vi "Main.vi"() -> ()   [LabVIEW 2019]
uses:
  <vilib>/vision/Image Controls.llb/IMAQ Image.ctl
  <vilib>/vision/NI_Vision_Development_Module.lvlib
panel:
  out "Otwarte":bool
  in  "Save Button":bool
  in  "Clear Button":bool
  in  "Image Path":path=path "D:/Krystian/Krystian/LabVIEW Data/OSP Projekt/Data/(0).jpg" caption="Picture Path"
  in  "Exit":bool
  in  "Start":bool
  out "Results":string
  out "Image":T1(plugin-control)
  # "Application Panel"
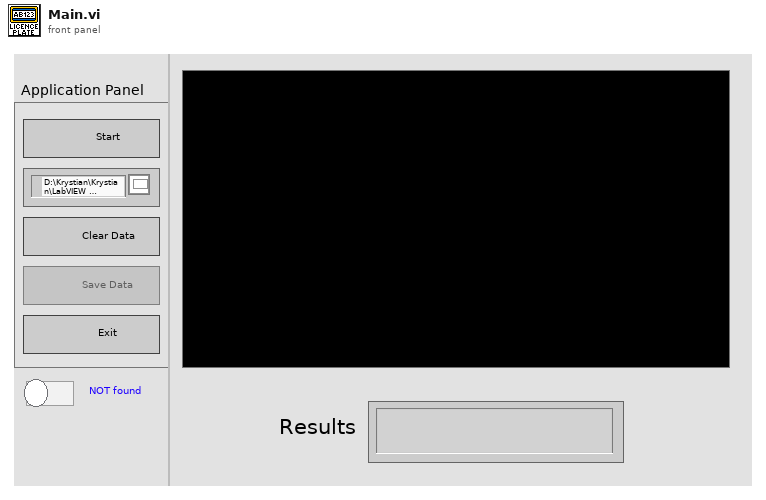
[diagram p1: front panel]
types:
  T1 = typedef "IMAQ Image.ctl" = refnum<image>
  T2 = enum32{"Invalid", "Standard", "Closed", "Hidden", "Minimized", "Maximized"}
  T3 = enum32{"invalid app kind", "Development System", "Run Time System", "Student Edition", "Embedded LabVIEW", "Evaluation", "Custom"}
  T4 = enum8{"Enabled", "Disabled", "Disabled and Grayed Out"}
  T5 = cluster{"Core":cluster{"Current VI Reference":refnum<vi>, "Close Panel on Exit?":bool}, "Save Button":refnum<vi>, "Results":string, "Image Path":path, "Data":cluster{"Rectangle":i32[]}, "Image":refnum<image>, "Python Path":path}
  T6 = cluster{"Current VI Reference":refnum<vi>, "Close Panel on Exit?":bool}
  T7 = typedef "Image Type" = u32
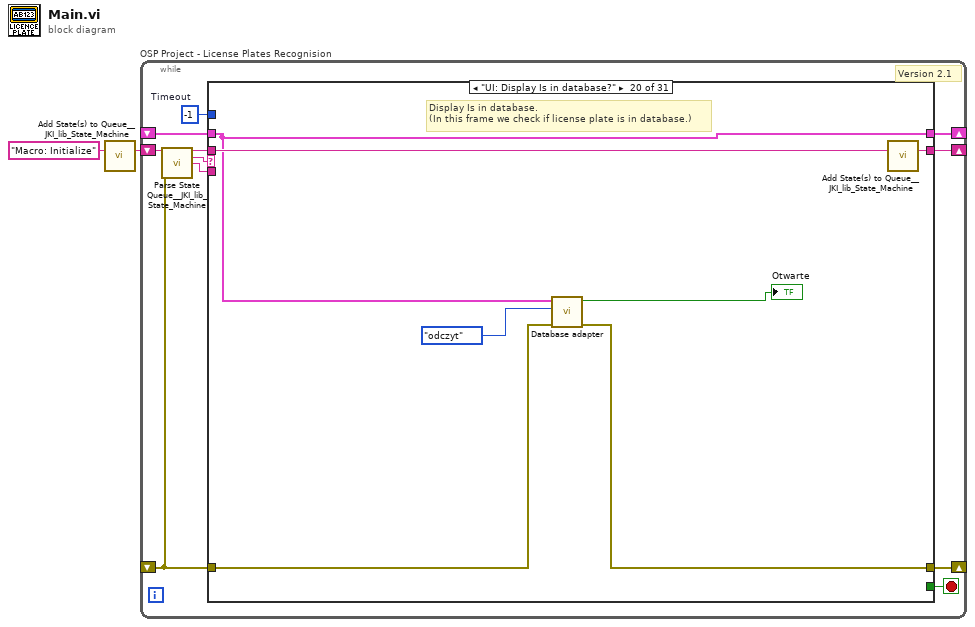
[diagram p0: block diagram]
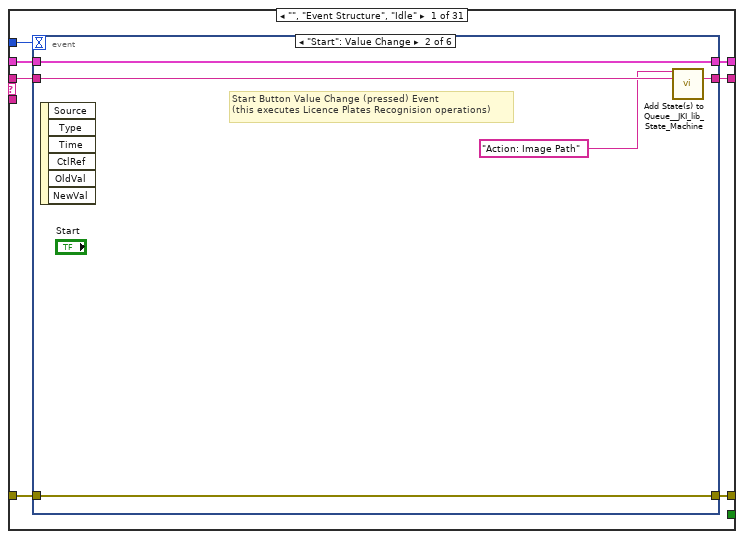
[diagram p2: hidden frame]
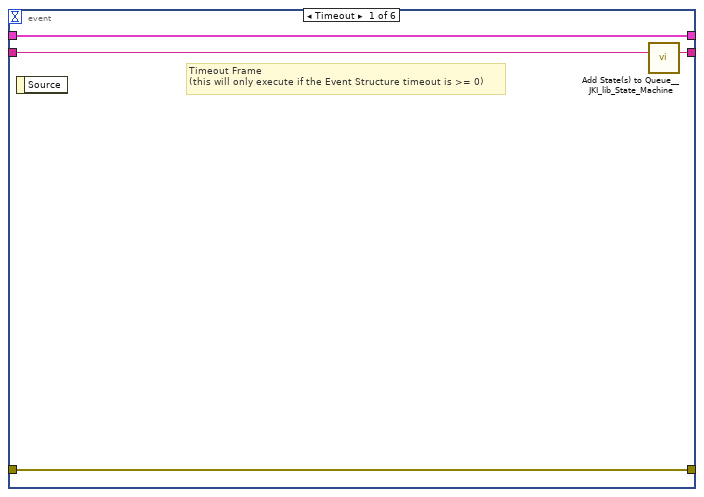
[diagram p3: hidden frame]
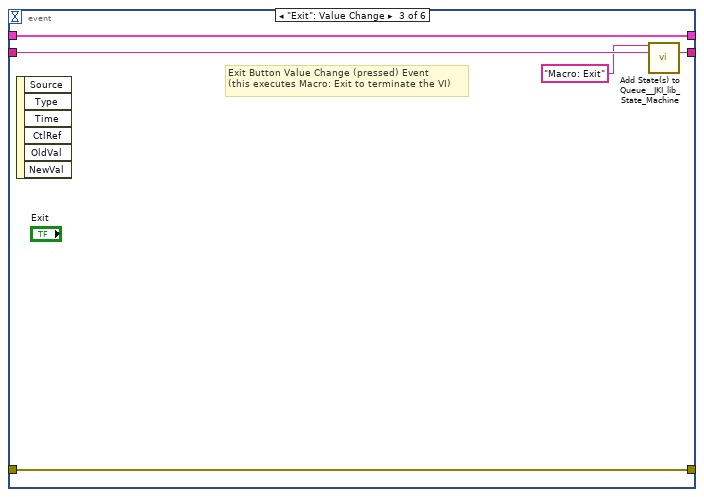
[diagram p4: hidden frame]
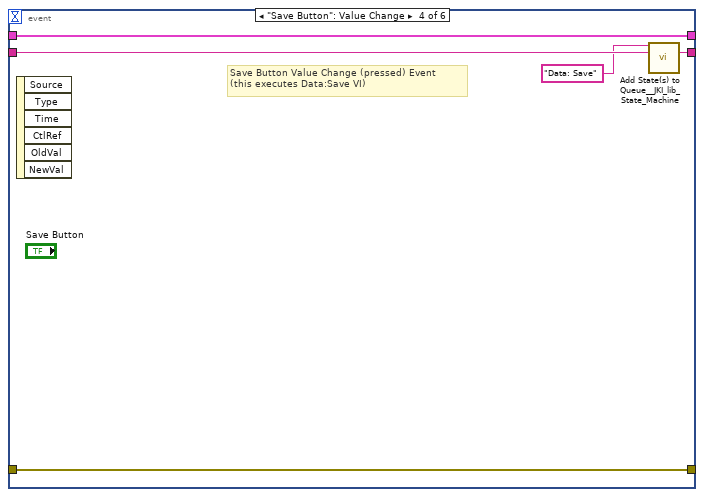
[diagram p5: hidden frame]
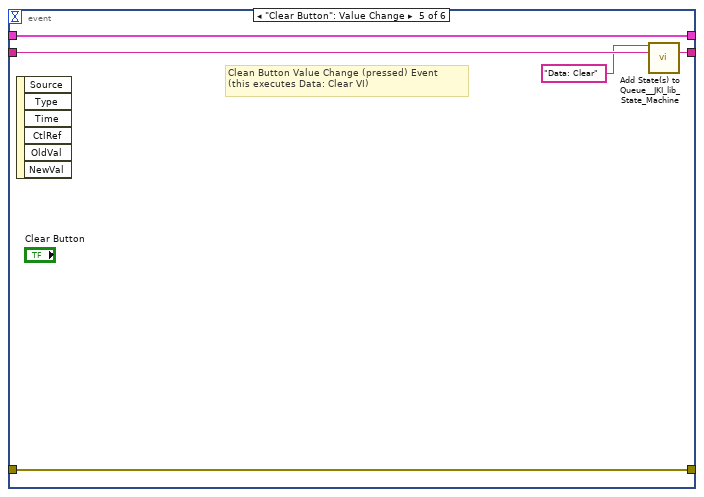
[diagram p6: hidden frame]
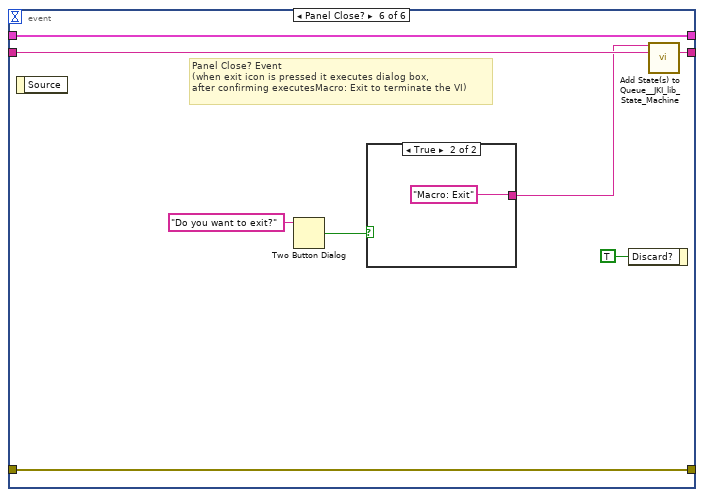
[diagram p7: hidden frame]
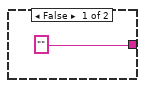
[diagram p8: hidden frame]
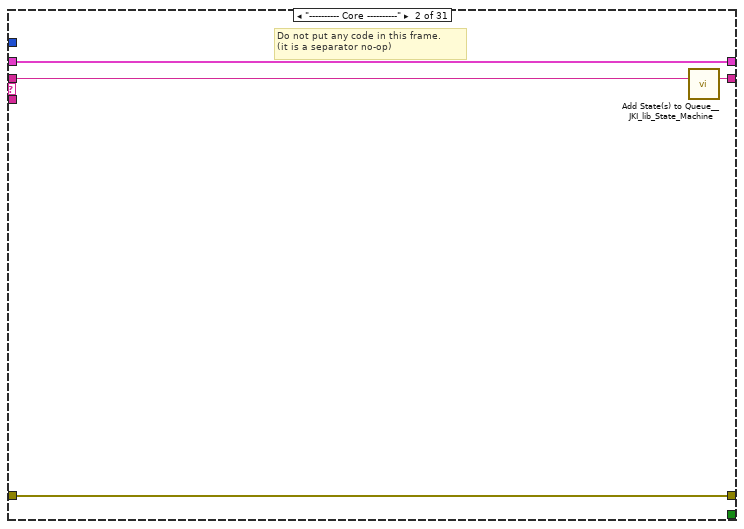
[diagram p9: hidden frame]
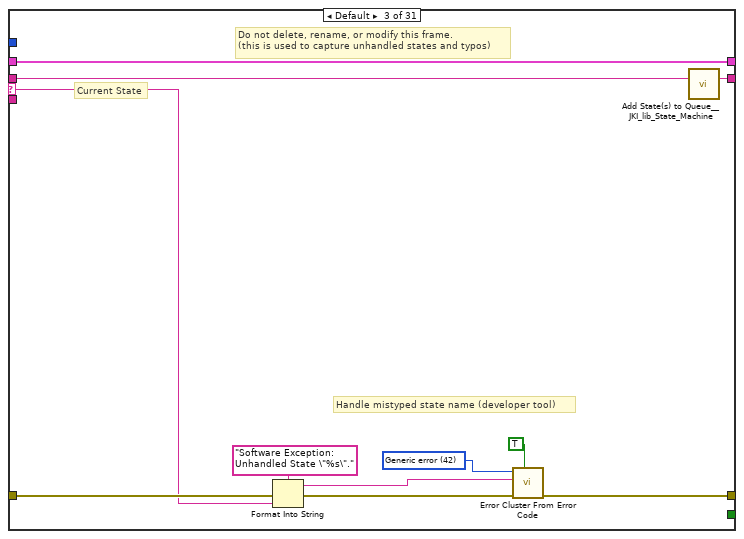
[diagram p10: hidden frame]
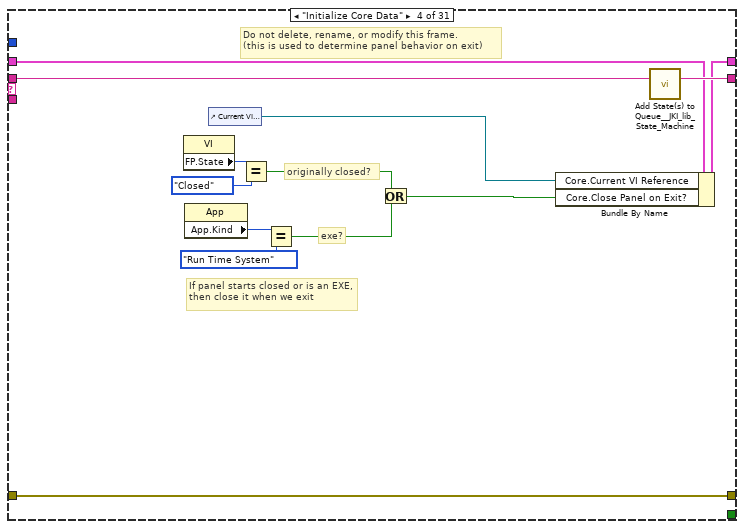
[diagram p11: hidden frame]
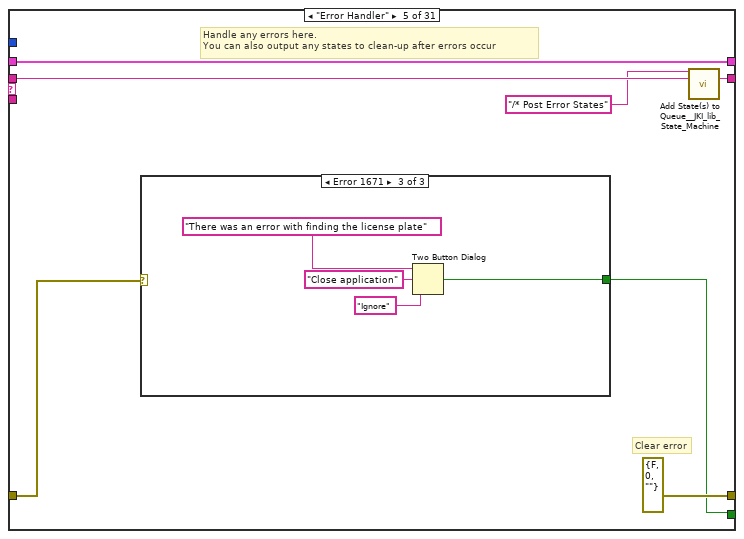
[diagram p12: hidden frame]
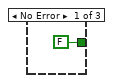
[diagram p13: hidden frame]
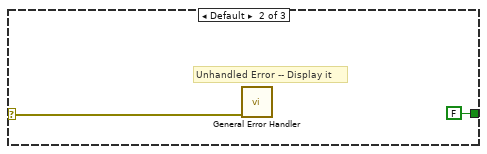
[diagram p14: hidden frame]
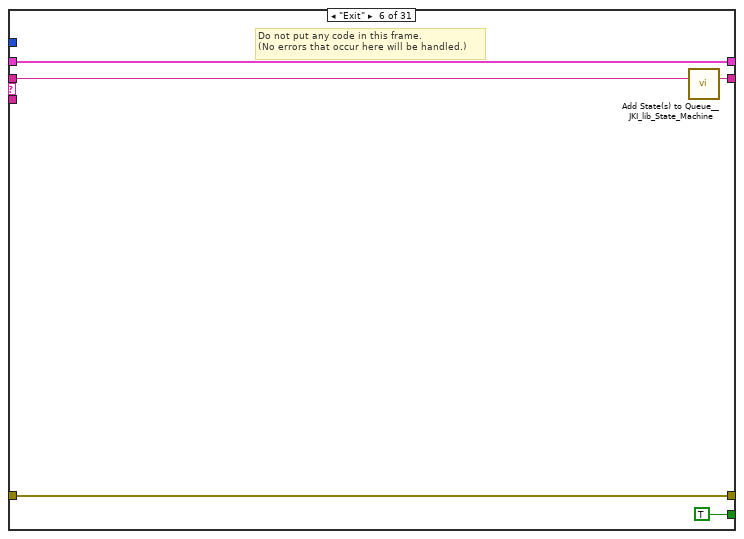
[diagram p15: hidden frame]
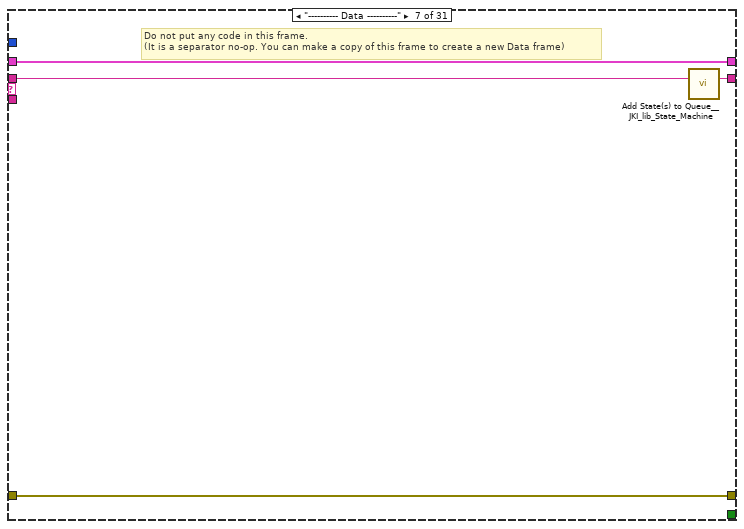
[diagram p16: hidden frame]
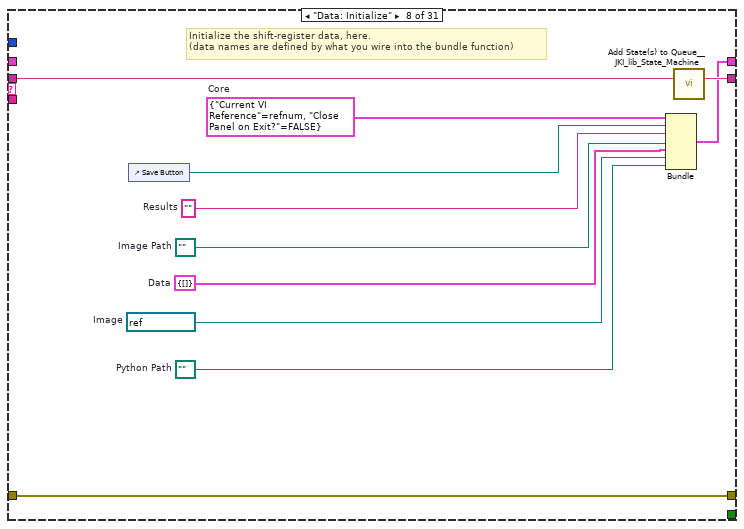
[diagram p17: hidden frame]
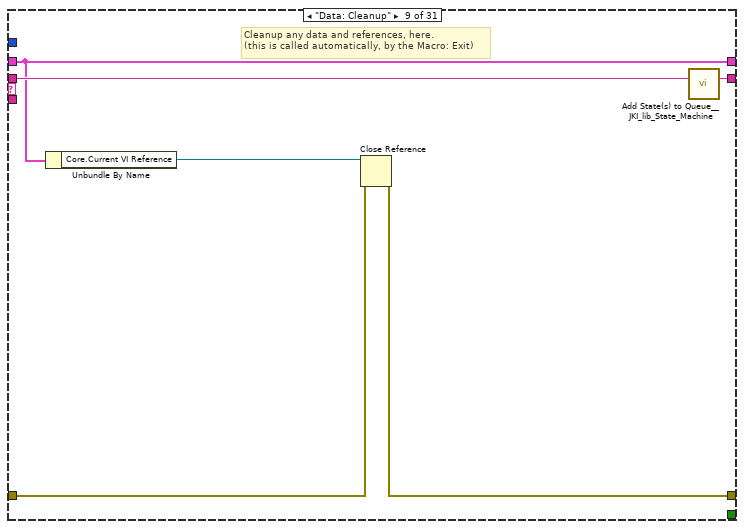
[diagram p18: hidden frame]
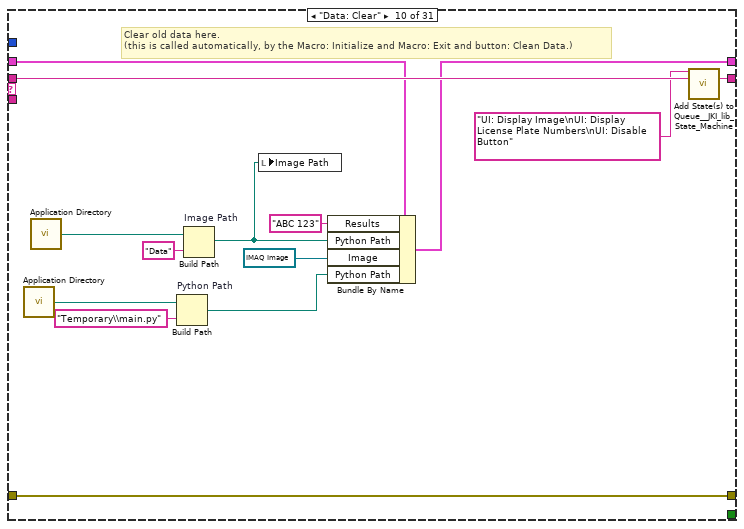
[diagram p19: hidden frame]
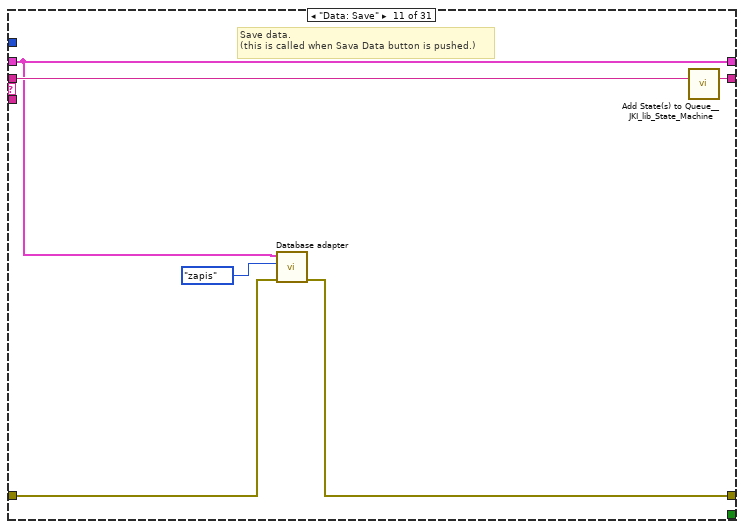
[diagram p20: hidden frame]
diagram:
  n1 = call <vilib>:"Add State(s) to Queue__JKI_lib_State_Machine.vi"("State(s) in (\"\")"="Macro: Initialize") -> ("States Out"=w2:string)  [unwired: 14 in]
  n2 = while "OSP Project - License Plates Recognision" {
    shift-right: [w6] -> _
    shift-left: _ -> [w5]
    shift-right: [w9] -> _
    shift-left: _ -> [w3]
    shift-right: [w8] -> _
    shift-left: w2 -> [w10]
    stop <- w7 stop-if-true
    w4 = -1  # Timeout
    # "Version 2.1"
    n3 = call <vilib>:"Parse State Queue__JKI_lib_State_Machine.vi"("State Queue"=w10, "Error In (no error)"=w3) -> ("Remaining States"=w12:string, "Current State"=w13:string, "Arguments"=w11:string)  [unwired: 11 in]
    n4 = case shown="\"UI: Display Is in database?\"" w13 {
      selector: w13 -> [_ _ w59 _ _ _ _ _ _ _ _ _ _ _ _ _ _ _ _ _ _ _ _ _ _ _ _ _ _ _ _]
      tunnel: w12 -> [w20 w58 w63 w82 w89 w101 w105 w116 w122 w136 w142 w146 w150 w156 w163 w169 w180 w250 w255 w262 w266 w271 w281 w285 w295 w325 w343 w353 w363 w375 w384]
      tunnel: w11 -> [_ _ _ _ _ _ _ _ _ _ _ _ _ _ _ w164 w174 _ _ _ _ _ _ _ _ _ _ _ _ _ _]
      tunnel: w5 -> [w18 w55 w61 w75 w86 w99 w102 _ w117 w132 w138 w143 w147 w153 w160 w167 w176 w247 w253 w258 w263 w268 w278 w282 w291 w310 w331 w350 w360 w368 w378]
      tunnel: [w17 w56 w65 w79 errorcluster {"status"=FALSE, "code"=0, "source"=""} ("error out") w98 w103 w113 w118 w134 w139 w144 w148 w154 w161 w165 w177 w248 w251 w260 w264 w269 w279 w283 w293 w313 w328 w344 w355 w365 w381] -> w9
      tunnel: w3 -> [w16 w56 w64 w79 w84 w98 w103 w113 w119 w134 w140 w144 w148 w154 w161 w166 w178 w248 w251 w259 w264 w269 w279 w283 w293 w314 w326 w345 w354 w364 w380]
      tunnel: [w19 w57 w62 w81 w88 w100 w104 w115 w121 w135 w141 w145 w149 w155 w162 w168 w179 w249 w254 w261 w265 w270 w280 w284 w294 w324 w342 w352 w362 w374 w383] -> w8
      tunnel: [_ _ _ _ w83 TRUE _ _ _ _ _ _ _ _ _ _ _ _ _ _ _ _ _ _ _ _ _ _ _ _ _] -> w7
      tunnel: [w15 w55 w61 w80 w86 w99 w102 w114 w117 w133 w138 w143 w147 w153 w160 w167 w176 w247 w253 w258 w263 w268 w278 w282 w292 w312 w332 w351 w361 w369 w379] -> w6
      tunnel: w4 -> [w14 _ _ _ _ _ _ _ _ _ _ _ _ _ _ _ _ _ _ _ _ _ _ _ _ _ _ _ _ _ _]
      frame "", "Event Structure", "Idle" {
        n5 = event shown="[1] \"Start\": Value Change" {
          selector: _ -> [_ _ _ _ _ _]
          dyn-events: _ -> [_ _ _ _ _ _]
          timeout: w14 -> [_ _ _ _ _ _]
          tunnel: w20 -> [w24 w29 w34 w39 w44 w52]
          tunnel: [w23 w28 w33 w38 w43 w51] -> w19
          tunnel: w18 -> [w21 w26 w31 w36 w41 w49]
          tunnel: [w22 w27 w32 w37 w42 w50] -> w17
          tunnel: w16 -> [w22 w27 w32 w37 w42 w50]
          tunnel: [w21 w26 w31 w36 w41 w49] -> w15
          event Timeout {
            # "Timeout Frame\n(this will only execute if the Event Structure timeout is >= 0)"
            n6 = event-data() -> ()  [unwired: 1 in, 1 out]
            n7 = call <vilib>:"Add State(s) to Queue__JKI_lib_State_Machine.vi"("State(s) in (\"\")"=w24) -> ("States Out"=w23:string)  [unwired: 14 in]
          }
          event "Start": Value Change {
            # "Start Button Value Change (pressed) Event\n(this executes Licence Plates Recognision operations)"
            n8 = event-data() -> ()  [unwired: 1 in, 6 out]
            n9 = call <vilib>:"Add State(s) to Queue__JKI_lib_State_Machine.vi"("State(s) in Front (\"\")"="Action: Image Path", "State(s) in (\"\")"=w29) -> ("States Out"=w28:string)  [unwired: 13 in]
          }
          event "Exit": Value Change {
            # "Exit Button Value Change (pressed) Event\n(this executes Macro: Exit to terminate the VI)"
            n10 = event-data() -> ()  [unwired: 1 in, 6 out]
            n11 = call <vilib>:"Add State(s) to Queue__JKI_lib_State_Machine.vi"("State(s) in Front (\"\")"="Macro: Exit", "State(s) in (\"\")"=w34) -> ("States Out"=w33:string)  [unwired: 13 in]
          }
          event "Save Button": Value Change {
            # "Save Button Value Change (pressed) Event\n(this executes Data:Save VI)"
            n12 = event-data() -> ()  [unwired: 1 in, 6 out]
            n13 = call <vilib>:"Add State(s) to Queue__JKI_lib_State_Machine.vi"("State(s) in Front (\"\")"="Data: Save", "State(s) in (\"\")"=w39) -> ("States Out"=w38:string)  [unwired: 13 in]
          }
          event "Clear Button": Value Change {
            # "Clean Button Value Change (pressed) Event\n(this executes Data: Clear VI)"
            n14 = event-data() -> ()  [unwired: 1 in, 6 out]
            n15 = call <vilib>:"Add State(s) to Queue__JKI_lib_State_Machine.vi"("State(s) in Front (\"\")"="Data: Clear", "State(s) in (\"\")"=w44) -> ("States Out"=w43:string)  [unwired: 13 in]
          }
          event Panel Close? {
            # "Panel Close? Event\n(when exit icon is pressed it executes dialog box, \nafter confirming executesMacro: Exit to terminate the VI)"
            n16 = event-data() -> ()  [unwired: 1 in, 1 out]
            n17 = Two Button Dialog(message="Do you want to exit?") -> (T button?=w47:bool)  [unwired: 2 in]
            n18 = case shown="True" w47 {
              tunnel: ["" "Macro: Exit"] -> w45
              frame False {
              }
              frame True {
              }
            }
            n19 = event-data("Discard?"=TRUE) -> ()  [unwired: 1 in, 1 out]
            n20 = call <vilib>:"Add State(s) to Queue__JKI_lib_State_Machine.vi"("State(s) in Front (\"\")"=w45, "State(s) in (\"\")"=w52) -> ("States Out"=w51:string)  [unwired: 13 in]
          }
        }
      }
      frame "---------- Core ----------" {
        # "Do not put any code in this frame.\n(it is a separator no-op)"
        n21 = call <vilib>:"Add State(s) to Queue__JKI_lib_State_Machine.vi"("State(s) in (\"\")"=w58) -> ("States Out"=w57:string)  [unwired: 14 in]
      }
      frame Default {
        w68 = 42 items=["No error", "Argument error", "Memory is full", "Out of zone", "End of file", "File already open", "Generic file I/O error", "File not found", "File permission error", "Disk is full", "Duplicate path", "Too many files open", "System feature not enabled", "Resource file not found", "Cannot add resource", "Resource not found", "Image not found", "Image memory error", "Pen does not exist", "Config type invalid", "Config token not found", "Config parse error", "Config memory error", "Bad external code format", "Bad external code offset", "External code not present", "Null window", "Destroy window error", "Null menu", "Print aborted", "Bad print record", "Print driver error", "Windows error during printing", "Memory error during printing", "Print dialog error", "Generic print error", "Invalid device refnum", "Device not found", "Device parameter error", "Device unit error", "Cannot open device", "Device call aborted", "Generic error", "Cancelled by user", "Object ID too low", "Object ID too high", "Object not in heap", "Unknown heap", "Unknown object (invalid DefProc)", "Unknown object (DefProc not in table)", "Message out of range", "Invalid (null) method", "Unknown message", "Manager call not supported", "Bad address", "Network operation in progress", "Network operation timed out", "Connection is busy", "Network attribute not supported", "Network error", "Address in use", "System out of memory", "Connection aborted", "Connection refused", "Not connected", "Already connected", "Connection closed", "Initialization error (interapplication manager)", "Bad occurrence", "Wait on unbound occurrence handler", "Occurrence queue overflow", "Datalog type conflict", "Unused", "Unrecognized type (interapplication manager)", "Memory corrupt", "Failed to make temporary DLL", "Old CIN version", "Drag socket not found", "Failed to load drop-object", "Failed to register OLE object", "Failed to release OLE object", "Format specifier type mismatch", "Unknown format specifier", "Too few format specifiers", "Too many format specifiers", "Scan failed", "Newer CIN version", "Error converting to variant", "Runtime menu error", "Password tampered", "Variant attribute not found", "Incompatible variant data type", "Event data is not available", "Event Store is not present", "Occurrence is not found", "Event Queue is not created", "Event info is not available", "Refnum passed is NULL", "Error retrieving Class GUID", "Error retrieving CoClass GUID", "Error retrieving TypeLib GUID.", "Bad built application magic bytes.", "Specific driver is different from the specific driver associated with the Logical Name.", "There is no session opened to the class driver.", "Max Error", "MAX - Error with config objects", "MAX - Error loading configuration", "MAX - Group not supported"]
        # "Current State"
        # "Do not delete, rename, or modify this frame.\n(this is used to capture unhandled states and typos)"
        # "Handle mistyped state name (developer tool)"
        n22 = Format Into String(format string="Software Exception: Unhandled State \"%s\"." ("message"), error in=w64, w59) -> (resulting string=w67:string, error out=w66:errorcluster)  [unwired: 1 in]
        n23 = call <vilib>:"Error Cluster From Error Code.vi"("show call chain? (False)"=TRUE, "error in (no error)"=w66, "error message (\"\")"=w67, "error code (0)"=w68) -> ("error out"=w65:errorcluster)  [unwired: 5 in]
        n24 = call <vilib>:"Add State(s) to Queue__JKI_lib_State_Machine.vi"("State(s) in (\"\")"=w63) -> ("States Out"=w62:string)  [unwired: 14 in]
      }
      frame "Initialize Core Data" {
        # "Do not delete, rename, or modify this frame.\n(this is used to determine panel behavior on exit)"
        # "originally closed?"
        # "exe?"
        # "If panel starts closed or is an EXE, then close it when we exit"
        n25 = property class="VI"() -> ("FP.State"=w72:T2)  [unwired: 2 in, 2 out]
        n26 = property class="App"() -> ("App.Kind"=w78:T3)  [unwired: 2 in, 2 out]
        n27 = control-ref of="Current VI Reference"() -> (w73:refnum<vi>)
        n28 = Equal?(x=w72, y=T2."Closed" ("Front Panel Window:State")) -> (x = y?=w70:bool)
        n29 = Equal?(x=w78, y=T3."Run Time System" ("Application:Kind")) -> (x = y?=w76:bool)
        n30 = Or(x=w70, y=w76) -> (x .or. y?=w74:bool)
        n31 = Bundle By Name(cluster=w75, "Core.Current VI Reference"=w73, "Core.Close Panel on Exit?"=w74) -> (w80:T5)
        n32 = call <vilib>:"Add State(s) to Queue__JKI_lib_State_Machine.vi"("State(s) in (\"\")"=w82) -> ("States Out"=w81:string)  [unwired: 14 in]
      }
      frame "Error Handler" {
        # "Handle any errors here.\nYou can also output any states to clean-up after errors occur"
        # "Clear error"
        n33 = case shown="Error 1671" w84 {
          selector: w84 -> [_ w91 _]
          tunnel: [FALSE ("T button?") FALSE ("T button?") w95] -> w83
          frame No Error {
          }
          frame Default {
            # "Unhandled Error -- Display it"
            n34 = call <vilib>:"General Error Handler.vi"("error in (no error)"=w91) -> ()  [unwired: 10 in, 5 out]
          }
          frame Error {
            n35 = Two Button Dialog(message="There was an error with finding the license plate", 1:"Ignore" ("F button name (\"Cancel\")"), 2:"Close application" ("T button name (\"OK\")")) -> (T button?=w95:bool)
          }
        }
        n36 = call <vilib>:"Add State(s) to Queue__JKI_lib_State_Machine.vi"("State(s) in Front (\"\")"="/* Post Error States", "State(s) in (\"\")"=w89) -> ("States Out"=w88:string)  [unwired: 13 in]
      }
      frame "Exit" {
        # "Do not put any code in this frame.\n(No errors that occur here will be handled.)"
        n37 = call <vilib>:"Add State(s) to Queue__JKI_lib_State_Machine.vi"("State(s) in (\"\")"=w101) -> ("States Out"=w100:string)  [unwired: 14 in]
      }
      frame "---------- Data ----------" {
        # "Do not put any code in this frame.\n(It is a separator no-op. You can make a copy of this frame to create a new Data frame)"
        n38 = call <vilib>:"Add State(s) to Queue__JKI_lib_State_Machine.vi"("State(s) in (\"\")"=w105) -> ("States Out"=w104:string)  [unwired: 14 in]
      }
      frame "Data: Initialize" {
        w107 = path ""  # Python Path
        w108 = path ""  # Image Path
        w109 = refnum<image> refnum  # Image
        w110 = cluster{"Rectangle":i32[]} {"Rectangle"=[]}  # Data
        w111 = T6 {"Current VI Reference"=refnum, "Close Panel on Exit?"=FALSE}  # Core
        w112 = ""  # Results
        # "Initialize the shift-register data, here.\n(data names are defined by what you wire into the bundle function)"
        n39 = control-ref of="Save Button"() -> (w106:refnum<vi>)
        n40 = Bundle("Core"=w111, "Save Button"=w106, "Results"=w112, "Image Path"=w108, "Data"=w110, "Image"=w109, "Python Path"=w107) -> (w114:T5)  [unwired: 1 in]
        n41 = call <vilib>:"Add State(s) to Queue__JKI_lib_State_Machine.vi"("State(s) in (\"\")"=w116) -> ("States Out"=w115:string)  [unwired: 14 in]
      }
      frame "Data: Cleanup" {
        # "Cleanup any data and references, here.\n(this is called automatically, by the Macro: Exit)"
        n42 = Unbundle By Name(w117) -> ("Core.Current VI Reference"=w120:refnum<vi>)
        n43 = Close Reference(reference=w120, error in (no error)=w119) -> (error out=w118:errorcluster)
        n44 = call <vilib>:"Add State(s) to Queue__JKI_lib_State_Machine.vi"("State(s) in (\"\")"=w122) -> ("States Out"=w121:string)  [unwired: 14 in]
      }
      frame "Data: Clear" {
        # "Clear old data here.\n(this is called automatically, by the Macro: Initialize and Macro: Exit and button: Clean Data.)"
        n45 = call <vilib>:"Application Directory.vi"() -> ("Application Directory"=w125:path)
        n46 = call <vilib>:"Application Directory.vi"() -> ("Application Directory"=w128:path)
        n47 = Build Path "Python Path"(base path=w125, name or relative path="Temporary\\main.py") -> (appended path=w123:path)
        n48 = Build Path "Image Path"(base path=w128, name or relative path="Data") -> (appended path=w126:path)
        n49 = local write "Image Path"(w126) -> ()
        n50 = Bundle By Name(cluster=w132, "Results"="ABC 123", "Python Path"=w126, "Image"=T1 refnum, "Python Path"=w123) -> (w133:T5)
        n51 = call <vilib>:"Add State(s) to Queue__JKI_lib_State_Machine.vi"("State(s) in Front (\"\")"="UI: Display Image\nUI: Display License Plate Numbers\nUI: Disable Button", "State(s) in (\"\")"=w136) -> ("States Out"=w135:string)  [unwired: 13 in]
      }
      frame "Data: Save" {
        # "Save data.\n(this is called when Sava Data button is pushed.)"
        n52 = call "Database adapter.vi"("error in (no error)"=w140, "Enum"=enum16{"odczyt", "zapis"}."zapis", "Cluster"=w138) -> ("error out"=w139:errorcluster)  [unwired: 6 in, 2 out]
        n53 = call <vilib>:"Add State(s) to Queue__JKI_lib_State_Machine.vi"("State(s) in (\"\")"=w142) -> ("States Out"=w141:string)  [unwired: 14 in]
      }
      frame "---------- UI ----------" {
        # "Do not put any code in this frame.\n(It is a separator no-op. You can make a copy of this frame to create a new UI frame)"
        n54 = call <vilib>:"Add State(s) to Queue__JKI_lib_State_Machine.vi"("State(s) in (\"\")"=w146) -> ("States Out"=w145:string)  [unwired: 14 in]
      }
      frame "UI: Initialize" {
        # "Initialize the User Interface, here.\n(this is called automatically, by the Macro: Init)"
        n55 = call <vilib>:"Add State(s) to Queue__JKI_lib_State_Machine.vi"("State(s) in (\"\")"=w150) -> ("States Out"=w149:string)  [unwired: 14 in]
      }
      frame "UI: Enable Button" {
        # "Enable Button.\n(In this frame save button is enabled.)"
        n56 = Unbundle By Name(w153) -> ("Save Button"=w152:refnum<vi>)
        n57 = property on="Property Node" class="Bool"(reference=w152, "DisabledEnum"=T4."Enabled" ("Disabled")) -> ()  [unwired: 1 in, 2 out]
        n58 = call <vilib>:"Add State(s) to Queue__JKI_lib_State_Machine.vi"("State(s) in (\"\")"=w156) -> ("States Out"=w155:string)  [unwired: 14 in]
      }
      frame "UI: Disable Button" {
        # "Disable Button.\n(In this frame save button is disabled and grayed out.)"
        n59 = Unbundle By Name(w160) -> ("Save Button"=w159:refnum<vi>)
        n60 = local write "Otwarte"(FALSE) -> ()
        n61 = property on="Property Node" class="Bool"(reference=w159, "DisabledEnum"=T4."Disabled and Grayed Out" ("Disabled")) -> ()  [unwired: 1 in, 2 out]
        n62 = call <vilib>:"Add State(s) to Queue__JKI_lib_State_Machine.vi"("State(s) in (\"\")"=w163) -> ("States Out"=w162:string)  [unwired: 14 in]
      }
      frame "UI: Cursor Set" {
        # "Argument"
        # "Set and Unset Cursor Busy.\n(Usage: \"UI: Cursor Set >> Busy|Idle\")"
        n63 = case shown="\"Idle\", Default" w164 {
          tunnel: w166 -> [w171 w173]
          tunnel: [w170 w172] -> w165
          frame "Idle", Default {
            n64 = call <vilib>:"Unset Busy.vi"("error in (no error)"=w171) -> ("error out"=w170:errorcluster)  [unwired: 10 in]
          }
          frame "Busy" {
            n65 = call <vilib>:"Set Busy.vi"("error in (no error)"=w173) -> ("error out"=w172:errorcluster)  [unwired: 9 in, 1 out]
          }
        }
        n66 = call <vilib>:"Add State(s) to Queue__JKI_lib_State_Machine.vi"("State(s) in (\"\")"=w169) -> ("States Out"=w168:string)  [unwired: 14 in]
      }
      frame "UI: Front Panel State" {
        # "Argument"
        # "Set Front Panel Open or Closed\n(Usage: \"UI: Front Panel State >> Open|Close\")"
        n67 = Unbundle By Name(w176) -> ("Core.Current VI Reference"=w175:refnum<vi>)
        n68 = case shown="\"Minimize\", \"Minimized\"" w174 {
          tunnel: w178 -> [w186 w201 w212 w225 w238]
          tunnel: [w188 w202 w214 w227 w240] -> w177
          tunnel: w175 -> [w187 w199 w213 w226 w239]
          frame "Open", "Standard", Default {
            w181 = T2."Standard" ("State")
            n69 = property class="VI"(reference=w187, error in=w186) -> (reference out=w184:refnum<vi>, error out=w185:errorcluster, "FP.State"=w183:T2)
            n70 = Not Equal?(x=w183, y=w181) -> (x != y?=w182:bool)
            n71 = case shown="True" w182 {
              tunnel: [w192 w194] -> w188
              tunnel: w185 -> [w191 w194]
              tunnel: w184 -> [w190 _]
              tunnel: w181 -> [w189 _]
              frame True {
                n72 = invoke class="VI" method="FP.Open"(reference=w190, error in=w191, "Activate"=TRUE, "State"=w189) -> (error out=w192:errorcluster)  [unwired: 1 in, 4 out]
              }
              frame False {
              }
            }
          }
          frame "Close", "Closed" {
            n73 = property class="VI"(reference=w199, error in=w201) -> (reference out=w198:refnum<vi>, error out=w200:errorcluster, "FP.State"=w196:T2)
            n74 = Not Equal?(x=w196, y=T2."Closed" ("Front Panel Window:State")) -> (x != y?=w195:bool)
            n75 = case shown="True" w195 {
              tunnel: [w203 w206] -> w202
              tunnel: w200 -> [w203 w205]
              tunnel: w198 -> [_ w204]
              frame False {
              }
              frame True {
                n76 = invoke class="VI" method="FP.Close"(reference=w204, error in=w205) -> (error out=w206:errorcluster)  [unwired: 1 in, 2 out]
              }
            }
          }
          frame "Hidden", "Hide" {
            w207 = T2."Hidden" ("State")
            n77 = property class="VI"(reference=w213, error in=w212) -> (reference out=w210:refnum<vi>, error out=w211:errorcluster, "FP.State"=w209:T2)
            n78 = Not Equal?(x=w209, y=w207) -> (x != y?=w208:bool)
            n79 = case shown="True" w208 {
              tunnel: [w218 w219] -> w214
              tunnel: w211 -> [w217 w219]
              tunnel: w210 -> [w216 _]
              tunnel: w207 -> [w215 _]
              frame True {
                n80 = invoke class="VI" method="FP.Open"(reference=w216, error in=w217, "State"=w215) -> (error out=w218:errorcluster)  [unwired: 2 in, 4 out]
              }
              frame False {
              }
            }
          }
          frame "Minimize", "Minimized" {
            w220 = T2."Minimized" ("State")
            n81 = property class="VI"(reference=w226, error in=w225) -> (reference out=w223:refnum<vi>, error out=w224:errorcluster, "FP.State"=w222:T2)
            n82 = Not Equal?(x=w222, y=w220) -> (x != y?=w221:bool)
            n83 = case shown="True" w221 {
              tunnel: [w231 w232] -> w227
              tunnel: w224 -> [w230 w232]
              tunnel: w223 -> [w229 _]
              tunnel: w220 -> [w228 _]
              frame True {
                n84 = invoke class="VI" method="FP.Open"(reference=w229, error in=w230, "State"=w228) -> (error out=w231:errorcluster)  [unwired: 2 in, 4 out]
              }
              frame False {
              }
            }
          }
          frame "Maximize", "Maximized" {
            w233 = T2."Maximized" ("State")
            n85 = property class="VI"(reference=w239, error in=w238) -> (reference out=w236:refnum<vi>, error out=w237:errorcluster, "FP.State"=w235:T2)
            n86 = Not Equal?(x=w235, y=w233) -> (x != y?=w234:bool)
            n87 = case shown="True" w234 {
              tunnel: [w244 w245] -> w240
              tunnel: w237 -> [w243 w245]
              tunnel: w236 -> [w242 _]
              tunnel: w233 -> [w241 _]
              frame True {
                n88 = invoke class="VI" method="FP.Open"(reference=w242, error in=w243, "State"=w241) -> (error out=w244:errorcluster)  [unwired: 2 in, 4 out]
              }
              frame False {
              }
            }
          }
        }
        n89 = call <vilib>:"Add State(s) to Queue__JKI_lib_State_Machine.vi"("State(s) in (\"\")"=w180) -> ("States Out"=w179:string)  [unwired: 14 in]
      }
      frame "UI: Display Image" {
        # "Display Image\n(In this frame Image is displayed on UI.)"
        n90 = Unbundle By Name(w247) -> ("Image"=→"Image":refnum<image>)
        n91 = call <vilib>:"Add State(s) to Queue__JKI_lib_State_Machine.vi"("State(s) in (\"\")"=w250) -> ("States Out"=w249:string)  [unwired: 14 in]
      }
      frame "UI: Display License Plate Numbers" {
        # "Display License Plate Numbers\n(In this frame Resoults are displayed on UI.)"
        n92 = Unbundle By Name(w253) -> ("Results"=→"Results":string)
        n93 = call <vilib>:"Add State(s) to Queue__JKI_lib_State_Machine.vi"("State(s) in (\"\")"=w255) -> ("States Out"=w254:string)  [unwired: 14 in]
      }
      frame "UI: Display Is in database?" {
        # "Display Is in database.\n(In this frame we check if license plate is in database.)"
        n94 = call "Database adapter.vi"("error in (no error)"=w259, "Enum"=enum16{"odczyt", "zapis"}."odczyt", "Cluster"=w258) -> ("error out"=w260:errorcluster, "Boolean"=→"Otwarte":bool)  [unwired: 6 in, 1 out]
        n95 = call <vilib>:"Add State(s) to Queue__JKI_lib_State_Machine.vi"("State(s) in (\"\")"=w262) -> ("States Out"=w261:string)  [unwired: 14 in]
      }
      frame "---------- Macro ----------" {
        # "Do not put any code in this frame.\n(It is a separator no-op. You can make a copy of this frame to create a new Macro frame)"
        n96 = call <vilib>:"Add State(s) to Queue__JKI_lib_State_Machine.vi"("State(s) in (\"\")"=w266) -> ("States Out"=w265:string)  [unwired: 14 in]
      }
      frame "Macro: Initialize" {
        w267 = "Data: Initialize\nInitialize Core Data\nData: Clear\nUI: Initialize\nUI: Disable Button\nUI: Front Panel State >> Open"  # Data: Initialize Initialize Core Data Data: Clear UI: Initialize UI: Disable Button UI: Front Panel State >> Open
        # "Initialization Macro\n(This is called once, when the VI starts)"
        n97 = call <vilib>:"Add State(s) to Queue__JKI_lib_State_Machine.vi"("State(s) in Front (\"\")"=w267, "State(s) in (\"\")"=w271) -> ("States Out"=w270:string)  [unwired: 13 in]
      }
      frame "Macro: Exit" {
        # "Exit Macro\n(This is called once, when the VI exits)"
        n98 = Unbundle By Name(w278) -> ("Core.Close Panel on Exit?"=w277:bool)
        n99 = Select(t="UI: Front Panel State >> Close", s=w277, f="") -> (s? t:f=w274:string)
        n100 = call <vilib>:"Add State(s) to Queue__JKI_lib_State_Machine.vi"("State(s) in (\"\")"=w274, "State(s) at Back (\"\")"="Data: Cleanup\nData: Clear\nExit") -> ("States Out"=w272:string)  [unwired: 13 in]
        n101 = call <vilib>:"Add State(s) to Queue__JKI_lib_State_Machine.vi"("State(s) in Front (\"\")"=w272, "State(s) in (\"\")"=w281) -> ("States Out"=w280:string)  [unwired: 13 in]
      }
      frame "---------- Action ----------" {
        # "Template Separator\n(You can make a copy of, or modify, this frame)"
        n102 = call <vilib>:"Add State(s) to Queue__JKI_lib_State_Machine.vi"("State(s) in (\"\")"=w285) -> ("States Out"=w284:string)  [unwired: 14 in]
      }
      frame "Action: Image Path" {
        w290 = path ""  # Empty Path Constant
        # "Image Path.\n(Checking if Image Path is correct.)"
        n103 = Equal?(x="Image Path", y=w290) -> (x = y?=w289:bool)
        n104 = case shown="True" w289 {
          tunnel: "Image Path" -> [w298 _]
          tunnel: [w299 TRUE] -> w286
          frame False {
            w300 = "jpg" ("search string/char (-)")
            n105 = Path To String(path=w298) -> (string=w301:string)
            n106 = Search/Split String(string=w301, search string/char (-)=w300) -> (match + rest of string=w302:string)  [unwired: 1 in, 2 out]
            n107 = Equal?(x=w302, y=w300) -> (x = y?=w299:bool)
          }
          frame True {
            n108 = One Button Dialog(message="Image path is EMPTY!\nPlease select image path.") -> ()  [unwired: 1 in, 1 out]
          }
        }
        n109 = Bundle By Name(cluster=w291, "Image Path"="Image Path") -> (w292:T5)
        n110 = case shown="False" w286 {
          tunnel: [_ "Action: Python Code"] -> w287
          frame False {
            n111 = One Button Dialog(message="Image path is NOT CORRECT!\nPlease select JPG image.") -> ()  [unwired: 1 in, 1 out]
          }
          frame True {
          }
        }
        n112 = call <vilib>:"Add State(s) to Queue__JKI_lib_State_Machine.vi"("State(s) in Front (\"\")"=w287, "State(s) in (\"\")"=w295) -> ("States Out"=w294:string)  [unwired: 13 in]
      }
      frame "Action: Python Code" {
        # "Python Code.\n(In this frame we are using Python Node to identify coordinates of license plate.)"
        n113 = Unbundle By Name(w310) -> ("Image Path"=w316:path)
        n114 = call <vilib>:"Application Directory.vi"() -> ("Application Directory"=w320:path)
        n115 = Path To String(path=w316) -> (string=w306:string)
        n116 = Build Path(base path=w320, name or relative path="Temporary\\dist\\main") -> (appended path=w308:path)
        n117 = Path To String(path=w308) -> (string=w307:string)
        n118 = Format Into String(format string="cmd /c %s\\\\main.exe %s " ("command line"), w307, w306) -> (resulting string=w305:string)  [unwired: 2 in, 1 out]
        n119 = call <vilib>:"System Exec.vi"("expected output size  (4096)"=u32 4096, "run minimized? (F)"=TRUE, "error in (no error)"=w314, "command line"=w305) -> ("error out"=w313:errorcluster, "standard output"=w321:string)  [unwired: 4 in, 2 out]
        n120 = call <userlib>:"String to 1D Array__ogtk.vi"("delimiter (Tab)"=",", "string"=w321) -> ("Array of Strings"=w323:string[])  [unwired: 9 in]
        n121 = Decimal String To Number(string=w323) -> (number=w322:i32[])  [unwired: 2 in, 1 out]
        n122 = Bundle By Name(cluster=w310, "Data.Rectangle"=w322) -> (w312:T5)
        n123 = call <vilib>:"Add State(s) to Queue__JKI_lib_State_Machine.vi"("State(s) in Front (\"\")"="Action: IMAQ Create" ("State(s) in Front (\"\")"), "State(s) in (\"\")"=w325) -> ("States Out"=w324:string)  [unwired: 13 in]
      }
      frame "Action: Python Code OLD" {
        w338 = "find_plate"  # function name
        w341 = "3.6"  # Python version
        # "Python Code.\n(In this frame we are using Python Node to identify coordinates of license plate.)"
        n124 = Unbundle By Name(w331) -> ("Image Path"=w334:path)
        n125 = Unbundle By Name(w331) -> ("Data.Rectangle"=w336:i32[])
        n126 = Unbundle By Name(w331) -> ("Python Path"=w335:path)
        n127 = Open Python Session(python version=w341, 3:w326) -> (session out=w340:refnum<k35>, error out=w327:errorcluster)  [unwired: 1 in]
        n128 = Path To String(path=w334) -> (string=w337:string)
        n129 = node(w340, w335, w338, w327, w336, w337) -> (w339:refnum<k35>, w329:errorcluster, w333:i32[])  [unwired: 1 in, 2 out]
        n130 = Close Python Session(session in=w339, error in=w329) -> (11:w328:errorcluster)
        n131 = Bundle By Name(cluster=w331, "Data.Rectangle"=w333) -> (w332:T5)
        n132 = call <vilib>:"Add State(s) to Queue__JKI_lib_State_Machine.vi"("State(s) in Front (\"\")"="Action: IMAQ Create" ("State(s) in Front (\"\")"), "State(s) in (\"\")"=w343) -> ("States Out"=w342:string)  [unwired: 13 in]
      }
      frame "Action: IMAQ Create" {
        w347 = T7 4 items=["Grayscale (U8)", "Grayscale (I16)", "Grayscale (SGL)", "Complex (CSG)", "RGB (U32)", "HSL (U32)", "RGB (U64)", "Grayscale (U16)"] ("Image Type")
        w348 = "untitled"  # Image Name
        # "IMAQ Create.\n(In this frame it is created a temorary memory location for an image.)"
        n133 = call "IMAQ Create"("Image Name"=w348, "Image Type"=w347, "error in (no error)"=w345) -> ("New Image"=w346:T1, "error out"=w344:errorcluster)  [unwired: 2 in]
        n134 = Bundle By Name(cluster=w350, "Image"=w346) -> (w351:T5)
        n135 = call <vilib>:"Add State(s) to Queue__JKI_lib_State_Machine.vi"("State(s) in Front (\"\")"="Action: IMAQ Read FIle" ("State(s) in Front (\"\")"), "State(s) in (\"\")"=w353) -> ("States Out"=w352:string)  [unwired: 13 in]
      }
      frame "Action: IMAQ Read FIle" {
        # "IMAQ Read File.\n(In this frame image file is being read.)"
        n136 = Unbundle By Name(w360) -> ("Image"=w357:refnum<image>)
        n137 = Unbundle By Name(w360) -> ("Image Path"=w358:path)
        n138 = call "IMAQ ReadFile 2"("File Path"=w358, "error in (no error)"=w354, "Image"=w357) -> ("error out"=w355:errorcluster, "Image Out"=w356:T1)  [unwired: 4 in, 3 out]
        n139 = Bundle By Name(cluster=w360, "Image"=w356) -> (w361:T5)
        n140 = call <vilib>:"Add State(s) to Queue__JKI_lib_State_Machine.vi"("State(s) in Front (\"\")"="Action: IMAQ Extract" ("State(s) in Front (\"\")"), "State(s) in (\"\")"=w363) -> ("States Out"=w362:string)  [unwired: 13 in]
      }
      frame "Action: IMAQ Extract" {
        w366 = 1  # Y Step Size
        w372 = 1  # X Step Size
        # "IMAQ Extract.\n(In this frame part of image is extracted with adjustment of the horizontal and vertical resolution.)"
        n141 = Unbundle By Name(w368) -> ("Data.Rectangle"=w371:i32[])
        n142 = Unbundle By Name(w368) -> ("Image"=w373:refnum<image>)
        n143 = call "IMAQ Extract 2"("Y Step Size"=w366, "Optional Rectangle"=w371, "error in (no error)"=w364, "X Step Size"=w372, "Image Src"=w373) -> ("error out"=w365:errorcluster, "Image Dst Out"=w370:T1)  [unwired: 5 in]
        n144 = Bundle By Name(cluster=w368, "Image"=w370) -> (w369:T5)
        n145 = call <vilib>:"Add State(s) to Queue__JKI_lib_State_Machine.vi"("State(s) in Front (\"\")"="UI: Display Image\nAction: IMAQ OCR", "State(s) in (\"\")"=w375) -> ("States Out"=w374:string)  [unwired: 13 in]
      }
      frame "Action: IMAQ OCR" {
        # "IMAQ OCR.\n(In this frame the optical character recognition is being used.)"
        n146 = Unbundle By Name(w378) -> ("Image"=w382:refnum<image>)
        n147 = call "IMAQ OCR.vi"("Image In"=w382, "error in"=w380) -> ("String (OCR/OCV 2)"=w377:string, "error out"=w381:errorcluster)  [unwired: 24 in]
        n148 = Bundle By Name(cluster=w378, "Results"=w377) -> (w379:T5)
        n149 = call <vilib>:"Add State(s) to Queue__JKI_lib_State_Machine.vi"("State(s) in Front (\"\")"="UI: Display License Plate Numbers\nUI: Enable Button\nUI: Display Is in database?" ("State(s) in Front (\"\")"), "State(s) in (\"\")"=w384) -> ("States Out"=w383:string)  [unwired: 13 in]
      }
    }
  }
